vi "MAIN Project.vi"() -> ()   [LabVIEW 2018]
doc: "Use this template to build a standard state machine design pattern. Each state executes code and determines which state to transition to. Contrast this design pattern with the User Interface Event Handler pattern, in which code executes in response to user actions. Contrast this design pattern also with the Queued Message Handler pattern, in which each message handling code can queue zero or more new messages."
uses:
  FSM States Project.ctl
panel:
  out "Motoren":bool[](array[boolean])
  out "Timer":dbl
  out "Current State":T1
  out "State to Recover from":T1
  in  "EMERGENCY":bool
  in  "ON/OFF":bool
  # "moet nog gewijzigd worden zodat \nmet behulp van een schakelaar de \ncount kan bijgehouden worden"
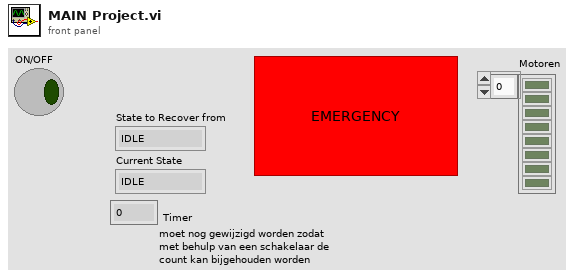
[diagram p1: front panel]
types:
  T1 = typedef "FSM States Project.ctl" = enum16{"IDLE", "EMERGENCY", "MOVE DOWNWARDS", "GRAB", "MOVE UPWARDS", "ROTATE", "DROP", "RETURN"}
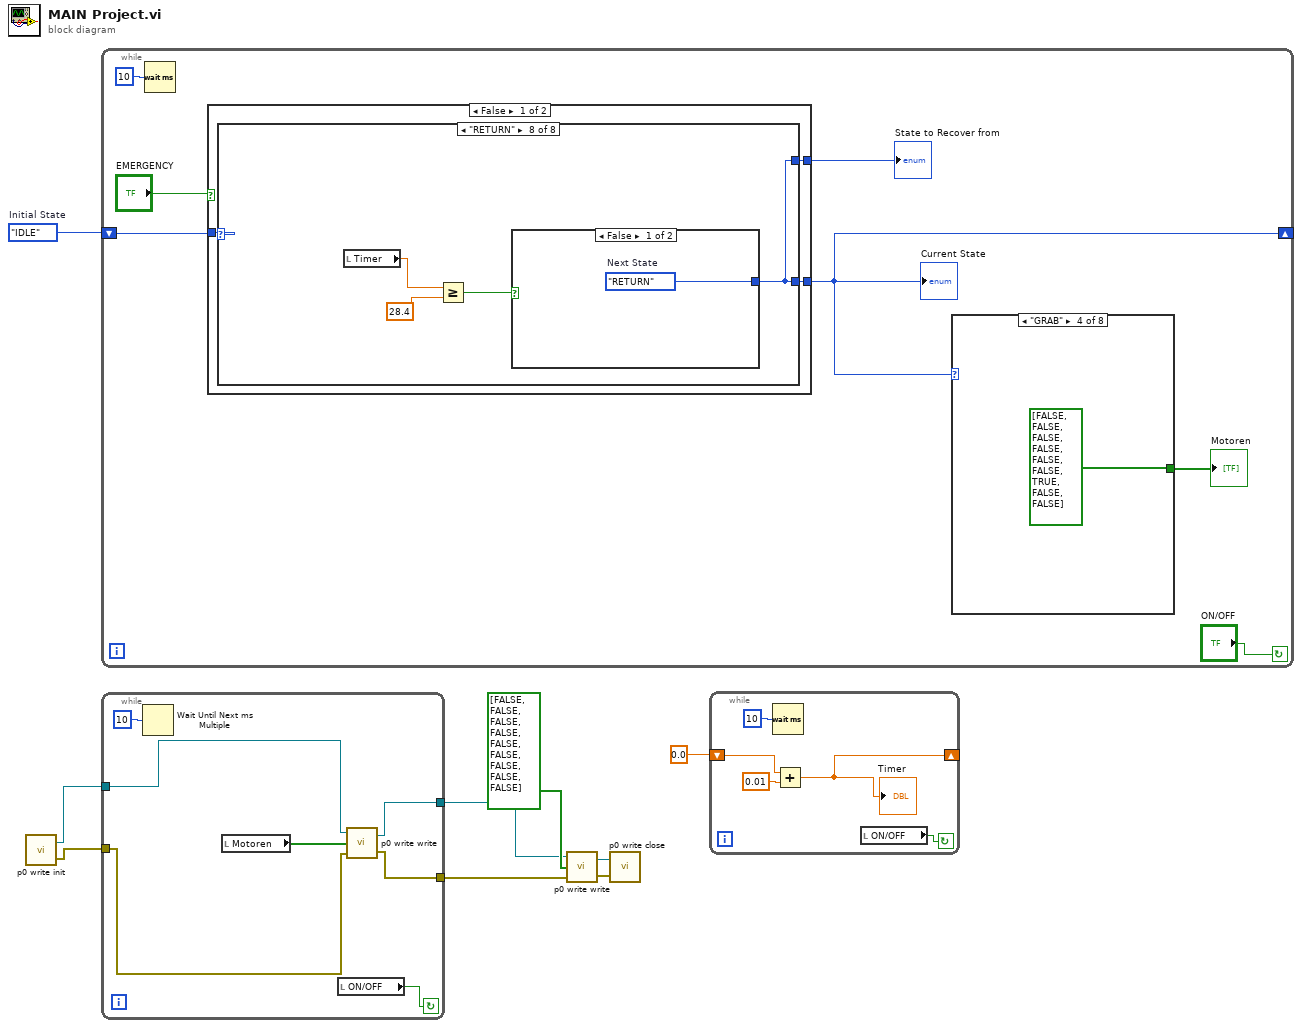
[diagram p0: block diagram]
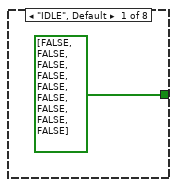
[diagram p2: hidden frame]
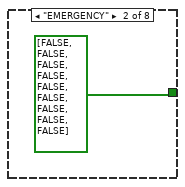
[diagram p3: hidden frame]
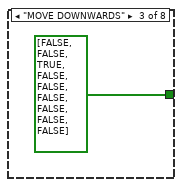
[diagram p4: hidden frame]
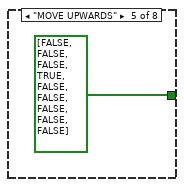
[diagram p5: hidden frame]
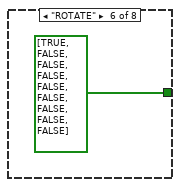
[diagram p6: hidden frame]
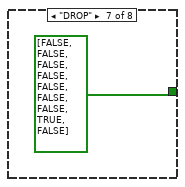
[diagram p7: hidden frame]
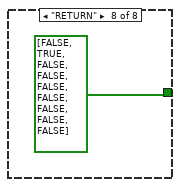
[diagram p8: hidden frame]
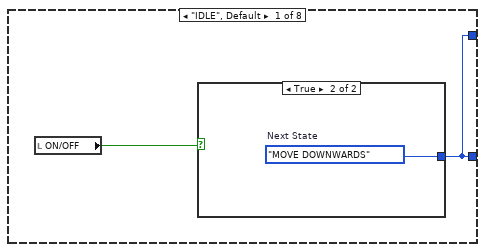
[diagram p9: hidden frame]
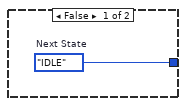
[diagram p10: hidden frame]
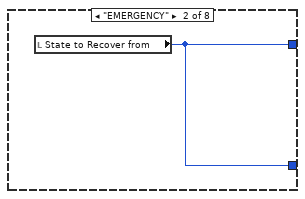
[diagram p11: hidden frame]
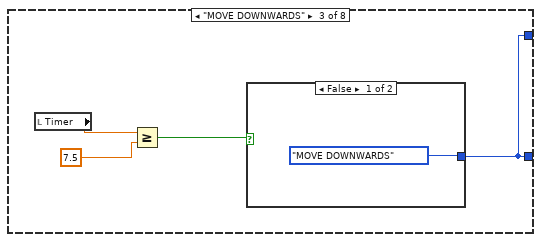
[diagram p12: hidden frame]
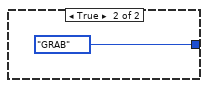
[diagram p13: hidden frame]
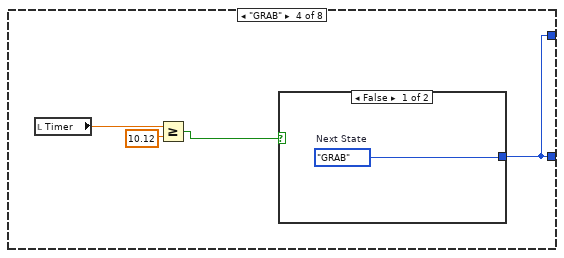
[diagram p14: hidden frame]
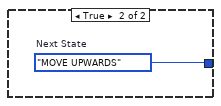
[diagram p15: hidden frame]
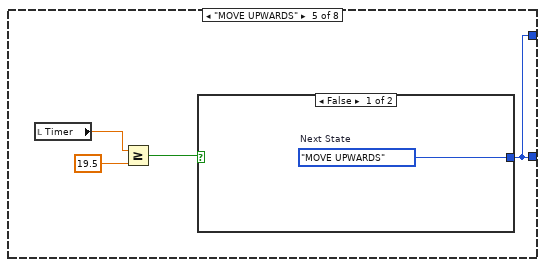
[diagram p16: hidden frame]
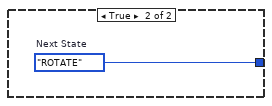
[diagram p17: hidden frame]
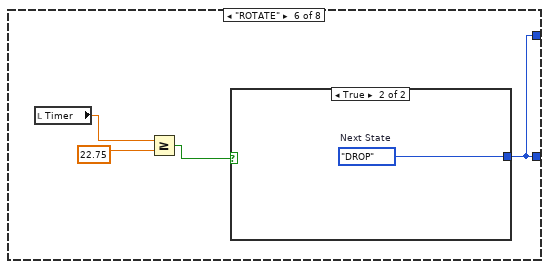
[diagram p18: hidden frame]
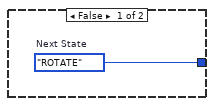
[diagram p19: hidden frame]
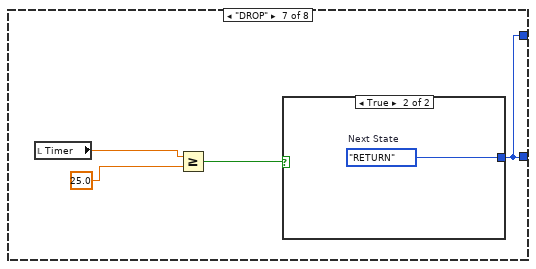
[diagram p20: hidden frame]
diagram:
  w9 = FSM_States_Project."IDLE"  # Initial State
  n1 = call "p0 write init.vi"() -> ("error out"=w3:errorcluster, "task out"=w2:refnum<k21>)
  n2 = while {
    shift-right: [w11] -> _
    shift-left: w9 -> [w14]
    stop <- "ON/OFF" continue-if-true
    n3 = Wait (ms)(milliseconds to wait=u32 10) -> ()  [unwired: 1 out]
    n4 = case shown="False" "EMERGENCY" {
      tunnel: w14 -> [w27 _]
      tunnel: [w25 w70] -> w13
      tunnel: [w26 FSM_States_Project."EMERGENCY" ("State to Recover from 2")] -> w11
      frame False {
        n5 = case shown="\"RETURN\"" w27 {
          tunnel: [w29 w32 w36 w39 w45 w54 w57 w66] -> w26
          tunnel: [w29 w32 w36 w39 w45 w54 w57 w66] -> w25
          frame "IDLE", Default {
            n6 = local read "ON/OFF"() -> (w28:bool)
            n7 = case shown="True" w28 {
              tunnel: [w30 w31] -> w29
              frame False {
                w30 = FSM_States_Project."IDLE"  # Next State
              }
              frame True {
                w31 = FSM_States_Project."MOVE DOWNWARDS"  # Next State
              }
            }
          }
          frame "EMERGENCY" {
            n8 = local read "State to Recover from"() -> (w32:T1)
          }
          frame "MOVE DOWNWARDS" {
            n9 = local read "Timer"() -> (w34:dbl)
            n10 = Greater Or Equal?(x=w34, y=7.5) -> (x >= y?=w35:bool)
            n11 = case shown="False" w35 {
              tunnel: [FSM_States_Project."MOVE DOWNWARDS" FSM_States_Project."GRAB"] -> w36
              frame False {
              }
              frame True {
              }
            }
          }
          frame "GRAB" {
            n12 = local read "Timer"() -> (w41:dbl)
            n13 = Greater Or Equal?(x=w41, y=10.12) -> (x >= y?=w42:bool)
            n14 = case shown="False" w42 {
              tunnel: [w43 w44] -> w39
              frame False {
                w43 = FSM_States_Project."GRAB"  # Next State
              }
              frame True {
                w44 = FSM_States_Project."MOVE UPWARDS"  # Next State
              }
            }
          }
          frame "MOVE UPWARDS" {
            n15 = local read "Timer"() -> (w48:dbl)
            n16 = Greater Or Equal?(x=w48, y=19.5) -> (x >= y?=w46:bool)
            n17 = case shown="False" w46 {
              tunnel: [w49 w50] -> w45
              frame False {
                w49 = FSM_States_Project."MOVE UPWARDS"  # Next State
              }
              frame True {
                w50 = FSM_States_Project."ROTATE"  # Next State
              }
            }
          }
          frame "ROTATE" {
            n18 = local read "Timer"() -> (w53:dbl)
            n19 = Greater Or Equal?(x=w53, y=22.75) -> (x >= y?=w51:bool)
            n20 = case shown="True" w51 {
              tunnel: [w55 w56] -> w54
              frame False {
                w55 = FSM_States_Project."ROTATE"  # Next State
              }
              frame True {
                w56 = FSM_States_Project."DROP"  # Next State
              }
            }
          }
          frame "DROP" {
            n21 = local read "Timer"() -> (w60:dbl)
            n22 = Greater Or Equal?(x=w60, y=25.0) -> (x >= y?=w58:bool)
            n23 = case shown="True" w58 {
              tunnel: [w61 w62] -> w57
              frame False {
                w61 = FSM_States_Project."DROP"  # Next State
              }
              frame True {
                w62 = FSM_States_Project."RETURN"  # Next State
              }
            }
          }
          frame "RETURN" {
            n24 = local read "Timer"() -> (w64:dbl)
            n25 = Greater Or Equal?(x=w64, y=28.4) -> (x >= y?=w65:bool)
            n26 = case shown="False" w65 {
              tunnel: [w67 w68] -> w66
              frame False {
                w67 = FSM_States_Project."RETURN"  # Next State
              }
              frame True {
                w68 = FSM_States_Project."IDLE"  # Next State
              }
            }
          }
        }
      }
      frame True {
        n27 = local read "State to Recover from"() -> (w70:T1)
      }
    }
    "State to Recover from" <- w13
    "Current State" <- w11
    n28 = case shown="\"GRAB\"" w11 {
      tunnel: [bool[] [FALSE, FALSE, FALSE, FALSE, FALSE, FALSE, FALSE, FALSE, FALSE] ("digital out") bool[] [FALSE, FALSE, FALSE, FALSE, FALSE, FALSE, FALSE, FALSE, FALSE] ("digital out") bool[] [FALSE, FALSE, TRUE, FALSE, FALSE, FALSE, FALSE, FALSE, FALSE] ("digital out") bool[] [FALSE, FALSE, FALSE, FALSE, FALSE, FALSE, TRUE, FALSE, FALSE] ("digital out") bool[] [FALSE, FALSE, FALSE, TRUE, FALSE, FALSE, FALSE, FALSE, FALSE] ("digital out") bool[] [TRUE, FALSE, FALSE, FALSE, FALSE, FALSE, FALSE, FALSE, FALSE] ("digital out") bool[] [FALSE, FALSE, FALSE, FALSE, FALSE, FALSE, FALSE, TRUE, FALSE] ("digital out") bool[] [FALSE, TRUE, FALSE, FALSE, FALSE, FALSE, FALSE, FALSE, FALSE] ("digital out")] -> w10
      frame "IDLE", Default {
      }
      frame "EMERGENCY" {
      }
      frame "MOVE DOWNWARDS" {
      }
      frame "GRAB" {
      }
      frame "MOVE UPWARDS" {
      }
      frame "ROTATE" {
      }
      frame "DROP" {
      }
      frame "RETURN" {
      }
    }
    "Motoren" <- w10
  }
  n29 = while {
    tunnel: [w76] -> w5
    tunnel: [w75] -> w4
    tunnel: w3 -> [w73]
    tunnel: w2 -> [w74]
    stop <- w77 continue-if-true
    n30 = Wait Until Next ms Multiple(millisecond multiple=u32 10) -> ()  [unwired: 1 out]
    n31 = local read "Motoren"() -> (w71:bool[])
    n32 = local read "ON/OFF"() -> (w77:bool)
    n33 = call "p0 write write.vi"("error in"=w73, "digital out"=w71, "task/channels in"=w74) -> ("error out"=w76:errorcluster, "task out"=w75:refnum<k21>)
  }
  n34 = call "p0 write write.vi"("error in"=w5, "digital out"=bool[] [FALSE, FALSE, FALSE, FALSE, FALSE, FALSE, FALSE, FALSE, FALSE], "task/channels in"=w4) -> ("error out"=w7:errorcluster, "task out"=w8:refnum<k21>)
  n35 = call "p0 write close.vi"("error in"=w7, "task/channels in"=w8) -> ()
  n36 = while {
    shift-right: [w78] -> _
    shift-left: 0.0 -> [w79]
    stop <- w82 continue-if-true
    n37 = Wait (ms)(milliseconds to wait=u32 10) -> ()  [unwired: 1 out]
    n38 = Add(x=w79, y=0.01) -> (x+y=w78:dbl)
    "Timer" <- w78
    n39 = local read "ON/OFF"() -> (w82:bool)
  }
